vi "set pane orgin.vi"(8 "error in":errorcluster) -> (0 "error out":errorcluster)   [LabVIEW 2023, in "Reusable Library.lvlib"]
doc: "This VI will set all the pane orgines of the caller VI to (0,0)"
uses:
  <vilib>/Utility/miscctls.llb/LVPointTypeDef.ctl
  Reusable Library.lvlib
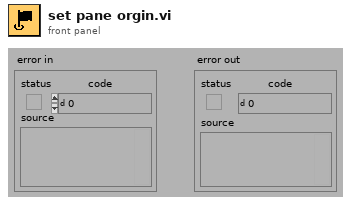
[diagram p1: front panel]
types:
  T1 = typedef "LVPointTypeDef.ctl" = cluster{"Horizontal":i16, "Vertical":i16}
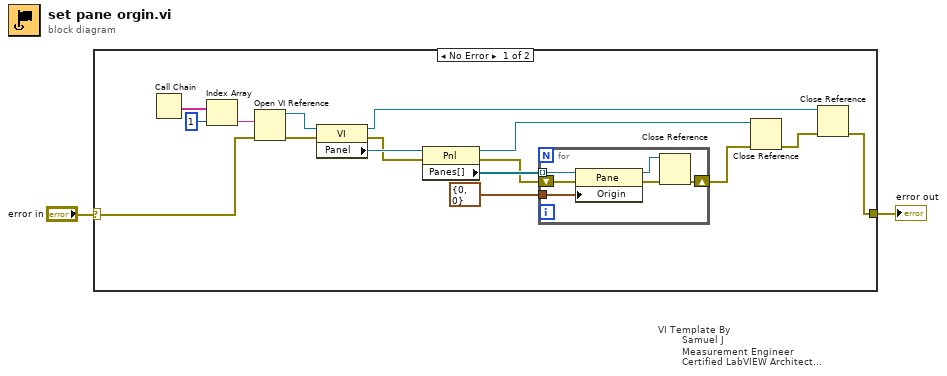
[diagram p0: block diagram]
diagram:
  n1 = case "VI Template By\n        Samuel J\n        Measurement Engineer\n        Certified LabVIEW Architect\n        Vestas Technology R&D, Chennai" shown="No Error" "error in" {
    selector: "error in" -> [w4 w25]
    tunnel: [w5 w25] -> w1
    frame No Error {
      n2 = Call Chain() -> (call chain=w18:string[])
      n3 = Index Array(array=w18, index=1) -> (element=w17:string)
      n4 = Open VI Reference(vi path=w17, error in (no error)=w4) -> (vi reference=w16:refnum<vi>, error out=w15:errorcluster)  [unwired: 4 in]
      n5 = property class="VI"(reference=w16, error in=w15) -> (reference out=w6:refnum<vi>, error out=w13:errorcluster, "Panel"=w14:refnum<vi>)
      n6 = property class="Pnl"(reference=w14, error in=w13) -> (reference out=w10:refnum<vi>, error out=w8:errorcluster, "Panes[]"=w12:refnum<vi>[])
      n7 = for {
        tunnel: w12 -> [w24] mode=indexing
        tunnel: T1 {"Horizontal"=0, "Vertical"=0} ("Origin") -> [w23]
        shift-right: [w20] -> w9
        shift-left: w8 -> [w19]
        n8 = property class="Pane"(reference=w24, error in=w19, "Origin"=w23) -> (reference out=w21:refnum<vi>, error out=w22:errorcluster)
        n9 = Close Reference(reference=w21, error in (no error)=w22) -> (error out=w20:errorcluster)
      }
      n10 = Close Reference(reference=w10, error in (no error)=w9) -> (error out=w7:errorcluster)
      n11 = Close Reference(reference=w6, error in (no error)=w7) -> (error out=w5:errorcluster)
    }
    frame Error {
    }
  }
  "error out" <- w1
